vi "INITIALIZE GROUP.vi"(8 "error in (no error)":errorcluster, 9 "Aceleração":dbl=3.0, 10 "Velocity":dbl=3.0, 11 "VISA Refnum in":refnum<visa-resource-name>) -> (0 "error out":errorcluster, 3 "VISA Refnum out":refnum<visa-resource-name>)   [LabVIEW 2014]
uses:
  <userlib>/Newport ESP301/Newport ESP301.lvlib
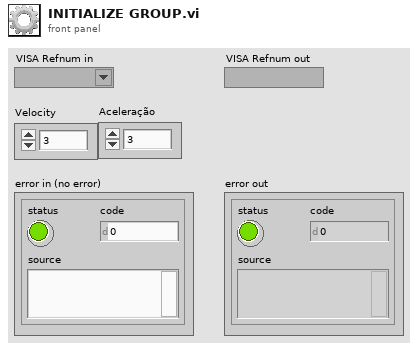
[diagram p1: front panel]
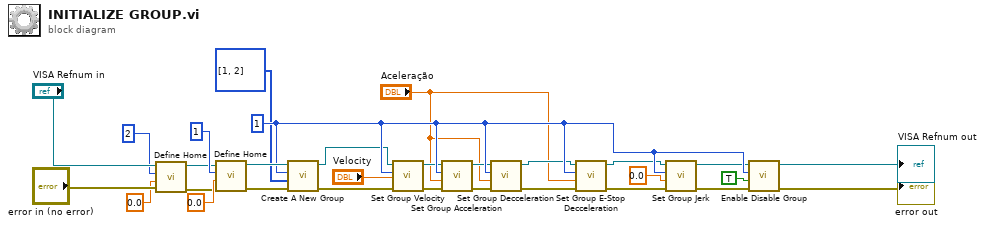
[diagram p0: block diagram]
diagram:
  w18 = 1 ("Group #")
  n1 = call <userlib>:"Define Home.vi"("error in (no error)"="error in (no error)", "Home Position (0 units)"=0.0, "Axis (1)"=2 ("y"), "VISA resource name"="VISA Refnum in") -> ("error out"=w20:errorcluster, "VISA resource name out"=w19:refnum<visa-resource-name>)  [unwired: 2 in]
  n2 = call <userlib>:"Define Home.vi"("error in (no error)"=w20, "Home Position (0 units)"=0.0, "Axis (1)"=1, "VISA resource name"=w19) -> ("error out"=w26:errorcluster, "VISA resource name out"=w25:refnum<visa-resource-name>)  [unwired: 2 in]
  n3 = call <userlib>:"Create A New Group.vi"("error in (no error)"=w26, "Axis Number"=i32[] [1, 2], "Group Number (1)"=w18, "VISA resource name"=w25) -> ("error out"=w4:errorcluster, "VISA resource name out"=w3:refnum<visa-resource-name>)  [unwired: 2 in]
  n4 = call <userlib>:"Set Group Velocity.vi"("error in (no error)"=w4, "Velocity (units/s)"="Velocity", "Group Number (1)"=w18, "VISA resource name"=w3) -> ("error out"=w9:errorcluster, "VISA resource name out"=w6:refnum<visa-resource-name>)  [unwired: 2 in]
  n5 = call <userlib>:"Set Group Acceleration.vi"("error in (no error)"=w9, "Acceleration (0 units/s²)"="Aceleração", "Group Number (1)"=w18, "VISA resource name"=w6) -> ("error out"=w8:errorcluster, "VISA resource name out"=w7:refnum<visa-resource-name>)  [unwired: 2 in]
  n6 = call <userlib>:"Set Group Decceleration.vi"("error in (no error)"=w8, "Decceleration (0 units/s²)"="Aceleração", "Group Number (1)"=w18, "VISA resource name"=w7) -> ("error out"=w13:errorcluster, "VISA resource name out"=w10:refnum<visa-resource-name>)  [unwired: 2 in]
  n7 = call <userlib>:"Set Group E-Stop Decceleration.vi"("error in (no error)"=w13, "E-Stop Decceleration (0 units/s²)"="Aceleração", "Group Number (1)"=w18, "VISA resource name"=w10) -> ("error out"=w14:errorcluster, "VISA resource name out"=w11:refnum<visa-resource-name>)  [unwired: 2 in]
  n8 = call <userlib>:"Set Group Jerk.vi"("error in (no error)"=w14, "Vector Jerk (0 units/s^3)"=0.0, "Group Number (1)"=w18, "VISA resource name"=w11) -> ("error out"=w15:errorcluster, "VISA resource name out"=w12:refnum<visa-resource-name>)  [unwired: 2 in]
  n9 = call <userlib>:"Enable Disable Group.vi"("error in (no error)"=w15, "Action (OFF)"=TRUE, "Group Number (1)"=w18, "VISA resource name"=w12) -> ("error out"=→"error out":errorcluster, "VISA resource name out"=→"VISA Refnum out":refnum<visa-resource-name>)  [unwired: 2 in]
